vi "Layout.vi"(0 "reference":refnum<class "ClassRelationshipEdge.lvclass">, 1 "graph":refnum<class "Graph.lvclass">, 2 "graphics":refnum<class "Graphics.lvclass">, 3 "grid":refnum<class "Grid.lvclass">, 5 "error in (no error)":errorcluster) -> (14 "reference out":refnum<class "ClassRelationshipEdge.lvclass">, 19 "error out":errorcluster)   [LabVIEW 2012, in "ClassRelationshipEdge.lvclass"]
uses:
  <resource>/Framework/Providers/Open_GDS/UML/ClassRelationshipEdge_class/ClassRelationshipEdge.lvclass
  <resource>/Framework/Providers/Open_GDS/UML/Grid_class/Grid.lvclass
  <resource>/Framework/Providers/Open_GDS/UML/Graphics_class/Graphics.lvclass
  <resource>/Framework/Providers/Open_GDS/UML/Graph_class/Graph.lvclass
  <resource>/Framework/Providers/Open_GDS/UML/BentStyle_class/BentStyle.lvclass
  <resource>/Framework/Providers/Open_GDS/UML/AbstractNode_class/AbstractNode.lvclass
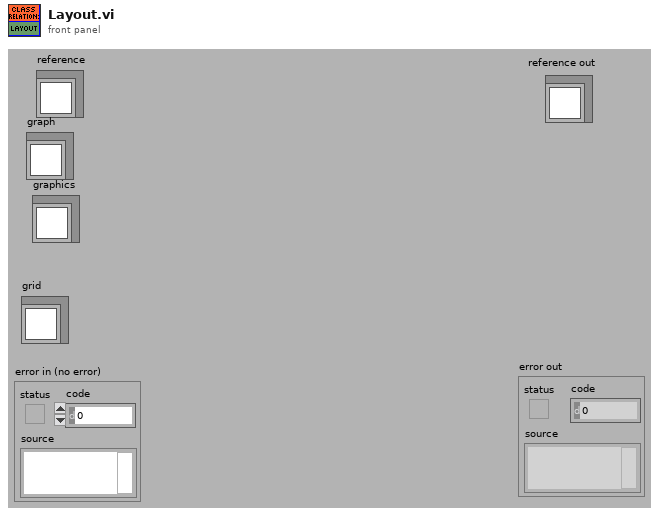
[diagram p1: front panel]
types:
  T1 = typedef "ClassRelationshipEdge.lvclass/ObjectAttributes.ctl" = cluster{"Base class":T2, "bentStyleRef":refnum<class "BentStyle.lvclass">, "startConnectionOffset":cluster{"x":i32, "y":i32}, "endConnectionOffset":cluster{"x":i32, "y":i32}, "MidLineOffset":cluster{"x":i32, "y":i32}, "DepClass":T6}
  T2 = typedef "SegmentedLineEdge.lvclass/ObjectAttributes.ctl" = cluster{"Base class":T3, "lineStyle":refnum<class "LineStyle.lvclass">, "startArrowHead":refnum<class "ArrowHead.lvclass">, "endArrowHead":refnum<class "ArrowHead.lvclass">, "startLabel":string, "midLabel":string, "endLabel":string, "MidLabelOffset":T5, "SplitWire":bool}
  T3 = typedef "GeneralPathEdge.lvclass/ObjectAttributes.ctl" = cluster{"Base class":T4}
  T4 = typedef "AbstractEdge.lvclass/ObjectAttributes.ctl" = cluster{"start":refnum<class "AbstractNode.lvclass">, "end":refnum<class "AbstractNode.lvclass">}
  T5 = typedef "Point Point2D.ctl" = cluster{"x":dbl, "y":dbl}
  T6 = typedef "ReversedEngineering_ViDependencyDetailsType.ctl" = cluster{"ThisVIs/Ctls":path[], "Dependent_VIs/Ctls":path[]}
  T7 = typedef "Rectangle Rectangle2D.ctl" = cluster{"x":dbl, "y":dbl, "width":dbl, "height":dbl}
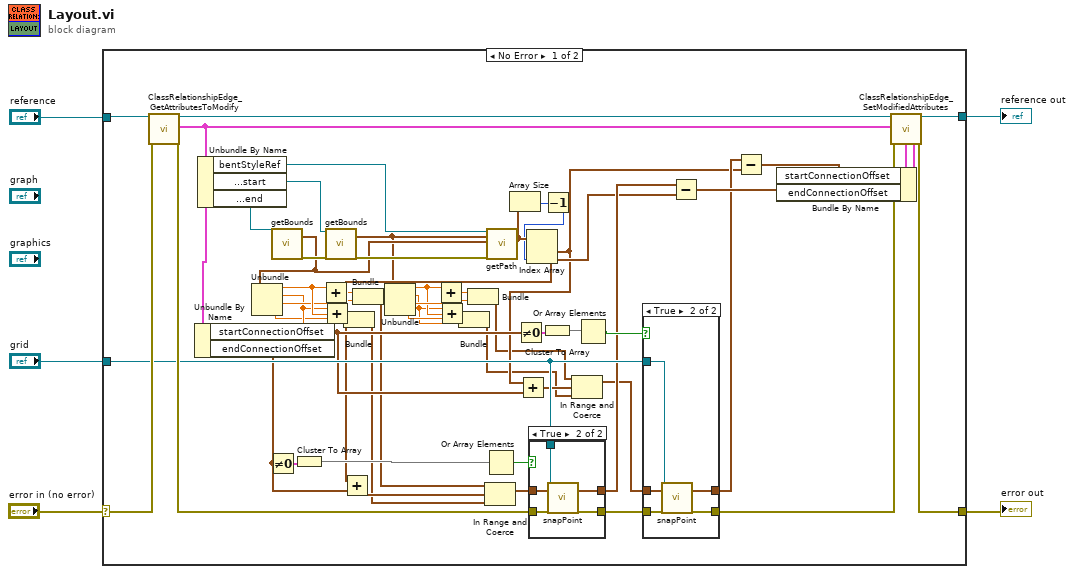
[diagram p0: block diagram]
diagram:
  n1 = case shown="No Error" "error in (no error)" {
    selector: "error in (no error)" -> [w60 w75]
    tunnel: "reference" -> [w59 w76]
    tunnel: [w56 w75] -> w3
    tunnel: [w55 w76] -> w2
    tunnel: "grid" -> [w50 _]
    frame No Error {
      n2 = call <resource>:"ClassRelationshipEdge_GetAttributesToModify.vi"("reference in"=w59, "error in (no error)"=w60) -> ("reference out"=w58:refnum<class "ClassRelationshipEdge.lvclass">, "Attributes"=w42:T1, "error out"=w54:errorcluster)  [unwired: 1 in, 14 out]
      n3 = Unbundle By Name(w42) -> ("startConnectionOffset"=w38:cluster{"x":i32, "y":i32}, "endConnectionOffset"=w37:cluster{"x":i32, "y":i32})
      n4 = Unbundle By Name(w42) -> ("bentStyleRef"=w39:refnum<class "BentStyle.lvclass">, "Base class.Base class.Base class.start"=w41:refnum<class "AbstractNode.lvclass">, "Base class.Base class.Base class.end"=w40:refnum<class "AbstractNode.lvclass">)
      n5 = Not Equal To 0?(x=w37) -> (x != 0?=w53:cluster{"x":bool, "y":bool})
      n6 = call-dynamic "getBounds.vi"("reference"=w40) -> ("bounds"=w23:T7, "error out"=w44:errorcluster)  [unwired: 1 in, 16 out]
      n7 = Unbundle(w23) -> ("x"=w22:dbl, "y"=w18:dbl, "width"=w21:dbl, "height"=w17:dbl)
      n8 = Cluster To Array(cluster=w53) -> (array=w52:bool[])
      n9 = Add(x=w22, y=w21) -> (x+y=w20:dbl)
      n10 = Add(x=w18, y=w17) -> (x+y=w19:dbl)
      n11 = call-dynamic "getBounds.vi"("reference"=w41, "error in (no error)"=w44) -> ("bounds"=w9:T7, "error out"=w43:errorcluster)  [unwired: 16 out]
      n12 = Bundle("x"=w22, "y"=w18) -> (w24:cluster{"x":dbl, "y":dbl})  [unwired: 1 out]
      n13 = Bundle(w20, w19) -> (w25:cluster{dbl, dbl})  [unwired: 1 out]
      n14 = Unbundle(w9) -> ("x"=w10:dbl, "y"=w8:dbl, "width"=w11:dbl, "height"=w14:dbl)
      n15 = Add(x=w10, y=w11) -> (x+y=w12:dbl)
      n16 = Add(x=w8, y=w14) -> (x+y=w13:dbl)
      n17 = Bundle("x"=w10, "y"=w8) -> (w6:cluster{"x":dbl, "y":dbl})  [unwired: 1 out]
      n18 = Bundle(w12, w13) -> (w7:cluster{dbl, dbl})  [unwired: 1 out]
      n19 = Or Array Elements(Boolean array=w52) -> (logical OR=w51:bool)
      n20 = call-dynamic "getPath.vi"("reference"=w39, "start"=w9, "end"=w23, "error in (no error)"=w43) -> ("path"=w30:T5[])  [unwired: 15 out]
      n21 = Array Size(array=w30) -> (size(s)=w29:i32)
      n22 = Not Equal To 0?(x=w38) -> (x != 0?=w48:cluster{"x":bool, "y":bool})
      n23 = Cluster To Array(cluster=w48) -> (array=w49:bool[])
      n24 = Decrement(x=w29) -> (x-1=w28:i32)
      n25 = Index Array(array=w30, index #2=w28) -> (element #1=w31:T5, element #2=w35:T5)  [unwired: 1 in]
      n26 = Add(x=w35, y=w37) -> (x+y=w27:T5)
      n27 = In Range and Coerce(upper limit=w25, x=w27, lower limit=w24) -> (coerced(x)=w26:T5)  [unwired: 1 out]
      n28 = Add(x=w31, y=w38) -> (x+y=w16:T5)
      n29 = case shown="True" w51 {
        tunnel: w54 -> [w68 w74]
        tunnel: w50 -> [_ w73]
        tunnel: w26 -> [w69 w72]
        tunnel: [w69 w71] -> w36
        tunnel: [w68 w70] -> w47
        frame False {
        }
        frame True {
          n30 = call <resource>:"snapPoint.vi"("reference"=w73, "point2D"=w72, "error in (no error)"=w74) -> ("point2D 2"=w71:T5, "error out"=w70:errorcluster)  [unwired: 15 out]
        }
      }
      n31 = In Range and Coerce(upper limit=w7, x=w16, lower limit=w6) -> (coerced(x)=w15:T5)  [unwired: 1 out]
      n32 = Or Array Elements(Boolean array=w49) -> (logical OR=w45:bool)
      n33 = case shown="True" w45 {
        tunnel: w47 -> [w61 w67]
        tunnel: w15 -> [w62 w66]
        tunnel: [w62 w65] -> w33
        tunnel: w50 -> [_ w64]
        tunnel: [w61 w63] -> w46
        frame False {
        }
        frame True {
          n34 = call <resource>:"snapPoint.vi"("reference"=w64, "point2D"=w66, "error in (no error)"=w67) -> ("point2D 2"=w65:T5, "error out"=w63:errorcluster)  [unwired: 15 out]
        }
      }
      n35 = Subtract(x=w36, y=w35) -> (x-y=w34:T5)
      n36 = Subtract(x=w33, y=w31) -> (x-y=w32:T5)
      n37 = Bundle By Name(cluster=w42, "startConnectionOffset"=w32, "endConnectionOffset"=w34) -> (w57:T1)
      n38 = call <resource>:"ClassRelationshipEdge_SetModifiedAttributes.vi"("reference in"=w58, "Attributes"=w57, "error in (no error)"=w46) -> ("reference out"=w55:refnum<class "ClassRelationshipEdge.lvclass">, "error out"=w56:errorcluster)  [unwired: 3 in, 12 out]
    }
    frame Error {
    }
  }
  "reference out" <- w2
  "error out" <- w3
